vi "write_dp_data.vi"(0 "dequeued data":dbl[][](array[numeric]), 1 "dP Data Labels":string[](array[string])=["Vap Mass Flow", "Liq Mass Flow", "DP", "Liq Tank P", "LiqTank T", "Sep P", "SepT", "Liq In P", "Liq In T", "Vap Tank P", "Vap Tank T", "Dev Section P", "Dev Section T", "Up TS P", "Up TS T", "Low TS P", "Low TS T", "Cond Top T", "Evap Top T", "Cond Bot T", "Evap Bot T", "Win 3-4 P", "Top Heat T", "Bot Heat T"], 2 "dP Data Index":dbl, 3 "dP Data Prefix":string, 4 "dP Data Folder":path) -> ()   [LabVIEW 2015]
uses:
  <vilib>/Utility/file.llb/Write Delimited Spreadsheet (DBL).vi
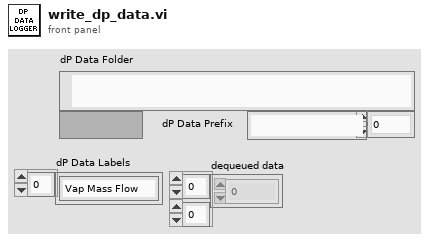
[diagram p1: front panel]
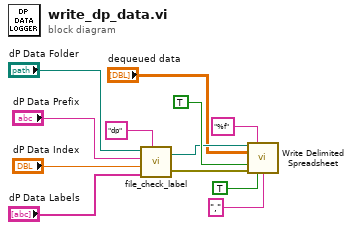
[diagram p0: block diagram]
diagram:
  n1 = call "file_check_label.vi"("base path"="dP Data Folder", "prefix"="dP Data Prefix", "index"="dP Data Index", "Loop Data Labels"="dP Data Labels", "task name"="dp") -> ("dup path"=w9:path, "error out"=w8:errorcluster)
  n2 = call-poly <vilib>:"Write Delimited Spreadsheet.vi"("file path (dialog if empty)"=w9, "format (%.3f)"="%f", "2D data"="dequeued data", "append to file? (new file:F)"=TRUE ("append to file? (F)"), "error in (no error)"=w8, "transpose? (no:F)"=TRUE ("transpose? (F)"), "delimiter (\\t)"="," ("delimiter (\\t)")) -> ()  [unwired: 7 in, 2 out]
